vi "MALT16PIN Output Get One.vi"(8 "error in":errorcluster, 9 "Port":i32=1, 10 "Address":i32) -> (0 "error out":errorcluster, 3 "status":bool)   [LabVIEW 2018, in "AltonTech MALT200817.lvlib"]
uses:
  <instrlib>/AltonTech MALT/AltonTech MALT200817.lvlib
  <instrlib>/AltonTech MALT/Public/Types/MALT Family Codes.ctl
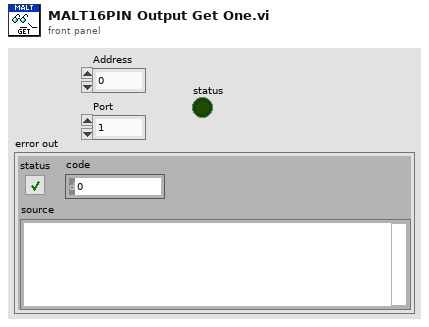
[diagram p1: front panel]
types:
  T1 = typedef "AltonTech MALT200817.lvlib/MALT Family Codes.ctl" = enum32{"-", "MALT40IO", "YAV904X8", "MALT132", "YAV91616", "MALT16PIN", "YAV90096", "YAV90HVT", "YAV90CLR", "YAV90128", "YAV90PNE", "YAVCANCON", "YAV91775", "YAV90XXX", "YAV90MMU", "H730050", "H710060", "H710061", "YAV90304", "MMI", "YAV90060", "MALT160T", "YAV90059", "Not Defined"}
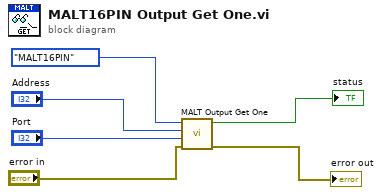
[diagram p0: block diagram]
diagram:
  n1 = call <instrlib>:"MALT Output Get One.vi"("error in"="error in", "Port"="Port", "Address"="Address", "MALT FamilyCode"=MALT_Family_Codes."MALT16PIN" ("MALT CardType")) -> ("error out"=→"error out":errorcluster, "Status"=→"status":bool)  [unwired: 6 in]
